vi "temp_FlpLib Ramp.vi"(0 "input":sgl, 1 "rampRate":sgl, 11 "stateIn":sgl format="%#_13g") -> (4 "output":sgl)   [LabVIEW 2016]
uses:
  <userlib>/_NI FLP Library/FPGA/outsideSCTL/FlpLib Add Shared Instance 0.vi
  <userlib>/_NI FLP Library/FPGA/outsideSCTL/FlpLib Subtract Shared Instance 0.vi
  <userlib>/_NI FLP Library/FPGA/outsideSCTL/FlpLib Greater Than Shared Instance 0.vi
  <userlib>/_NI FLP Library/FPGA/outsideSCTL/FlpLib Less Than Shared Instance 0.vi
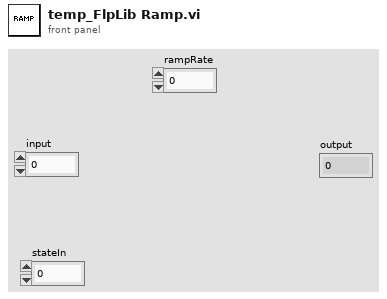
[diagram p1: front panel]
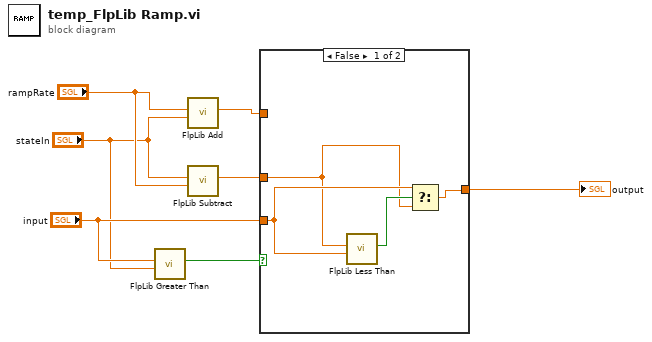
[diagram p0: block diagram]
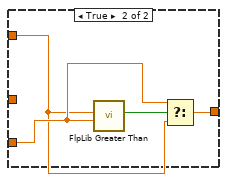
[diagram p2: hidden frame]
diagram:
  n1 = call-poly <userlib>:"FlpLib Greater Than.vi"("y"="stateIn", "x"="input") -> ("x > y?"=w6:bool)  [unwired: 5 in]
  n2 = call-poly <userlib>:"FlpLib Add.vi"("y"="stateIn", "x"="rampRate") -> ("x+y"=w1:sgl)  [unwired: 5 in]
  n3 = call-poly <userlib>:"FlpLib Subtract.vi"("y"="rampRate", "x"="stateIn") -> ("x-y"=w4:sgl)  [unwired: 5 in]
  n4 = case shown="False" w6 {
    tunnel: "input" -> [w9 w13]
    tunnel: [w10 w14] -> w5
    tunnel: w4 -> [w8 _]
    tunnel: w1 -> [_ w12]
    frame False {
      n5 = call-poly <userlib>:"FlpLib Less Than.vi"("y"=w9, "x"=w8) -> ("x < y?"=w11:bool)  [unwired: 5 in]
      n6 = Select(t=w9, s=w11, f=w8) -> (s? t:f=w10:sgl)
    }
    frame True {
      n7 = call-poly <userlib>:"FlpLib Greater Than.vi"("y"=w13, "x"=w12) -> ("x > y?"=w15:bool)  [unwired: 5 in]
      n8 = Select(t=w13, s=w15, f=w12) -> (s? t:f=w14:sgl)
    }
  }
  "output" <- w5
